vi "PH_Stepmotor_BaseClass.pack PSDB Data.vi"(0 "i ref in":refnum<vi>, 5 "error in (no error)":errorcluster) -> (14 "VI out":refnum<vi>, 15 "PSDB Boolean Data Array":T1[](array[typedef]), 17 "PSDB Numeric Data Array":T3[](array[typedef]), 18 "PSDB String Data Array":T2[](array[typedef]), 19 "error out":errorcluster)   [LabVIEW 2014, in "PH_Stepmotor_BaseClass.lvlib"]
uses:
  PH_Stepmotor_BaseClass.lvlib
  PH_Stepmotor_BaseClass.Motor Type.ctl
  PH_PSDBWriter/PH_PSDBWriter.Numeric dataset.ctl
  PH_PSDBWriter/PH_PSDBWriter.String dataset.ctl
  PH_PSDBWriter/PH_PSDBWriter.Boolean dataset.ctl
  PH_PSDBWriter/PH_PSDBWriter.lvlib
panel:
  in  "SW Scale.Motor Type":T4
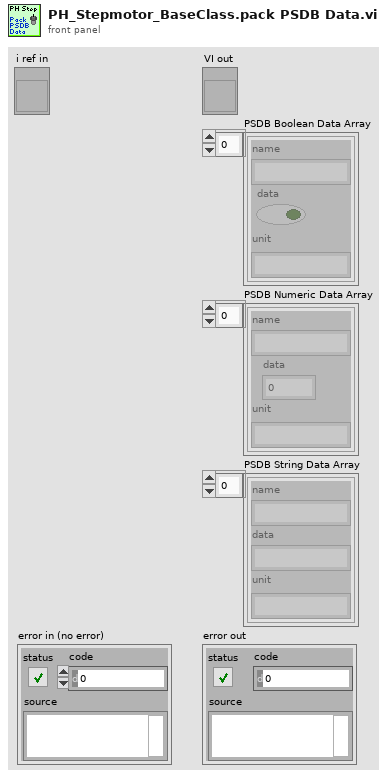
[diagram p1: front panel]
types:
  T1 = typedef "PH_PSDBWriter.lvlib/PH_PSDBWriter.Boolean dataset.ctl" = cluster{"name":string, "data":bool, "unit":string}
  T2 = typedef "PH_PSDBWriter.lvlib/PH_PSDBWriter.String dataset.ctl" = cluster{"name":string, "data":string, "unit":string}
  T3 = typedef "PH_PSDBWriter.lvlib/PH_PSDBWriter.Numeric dataset.ctl" = cluster{"name":string, "data":dbl, "unit":string}
  T4 = typedef "PH_Stepmotor_BaseClass.lvlib/PH_Stepmotor_BaseClass.Motor Type.ctl" = enum16{"Unspecific", "OWIS 49.120.2633", "OWIS 49.060.1033", "OWIS 43.040.2558", "Diamond Motion 2200 series", "OWIS 49.120.266B.MV6", "Calorimeter", "Linear Stage 1", "MICOS VT-80", "MICOS VT-80 S", "Standa Rotstage nt0.95A", "PUF RA 320.200", "PUF RA 800.200", "PUF RA 800.400", "PUF RA 400.50", "1324.nn.800.50", "1324.n9c.800.50", "1324.nn.320.200", "1324.nn.400.200", "1324.nn.800.200", "1324.nn.400.50", "1324.8c9c.800.50", "1324.8c9c.400.200"}
  T5 = typedef "PH_Stepmotor_BaseClass.lvlib/PH_Stepmotor_BaseClass.i attribute.ctl" = cluster{"Device Error":errorcluster, "Axes PSDB Thread":cluster{"Ref":refnum<vi>, "Q-Ref":refnum<queue>, "Data Status":T6}, "Axes":T7[], "Axes PSDB Infos":cluster{"GUI Name":string, "PSDB Instance ID":i32, "PSDB Status Service ID":i32, "Axis":i32, "Class":string}[], "GUI Refs":T11}
  T6 = typedef "PH_PSDBWriter.lvlib/PH_PSDBWriter.Data Status.ctl" = i16
  T7 = typedef "PH_Stepmotor_BaseClass.lvlib/PH_Stepmotor_BaseClass.Axis Attributes.ctl" = cluster{"Settings":T8, "Endswitch?":bool, "DIM Service IDs":T9, "Activity":T10, "Configured?":bool, "Position":cluster{"Current":i32, "Target":i32}, "Position to set":cluster{"New?":bool, "Wanted":i32}, "Stop?":bool, "Reset?":bool, "Move?":bool, "Nothing connected?":bool}
  T8 = typedef "PH_Stepmotor_BaseClass.lvlib/PH_Stepmotor_BaseClass.Axis Settings.ctl" = cluster{"Sign change":bool, "Width":dbl, "Calibration":dbl, "Unit":string, "Motor Type":T4, "Unit Width":string, "Unit CF":string}
  T9 = typedef "PH_Stepmotor_BaseClass.lvlib/PH_Stepmotor_BaseClass.Axis DIM Service IDs.ctl" = cluster{"Settings":i32, "Information":i32}
  T10 = typedef "PH_Stepmotor_BaseClass.lvlib/PH_Stepmotor_BaseClass.Axis Activity.ctl" = enum16{"No Information", "stopped", "running", "Failure", "Alarm", "stopped at backward ES", "stopped at foreward ES"}
  T11 = typedef "PH_Stepmotor_BaseClass.lvlib/PH_Stepmotor_BaseClass.GUI Refs.ctl" = cluster{"Axes Configuration":refnum<vi>, "Device Error":refnum<vi>, "Axes PSDB Infos":refnum<vi>}
  T12 = cluster{"GUI Name":string, "PSDB Instance ID":i32, "PSDB Status Service ID":i32, "Axis":i32, "Class":string}[]
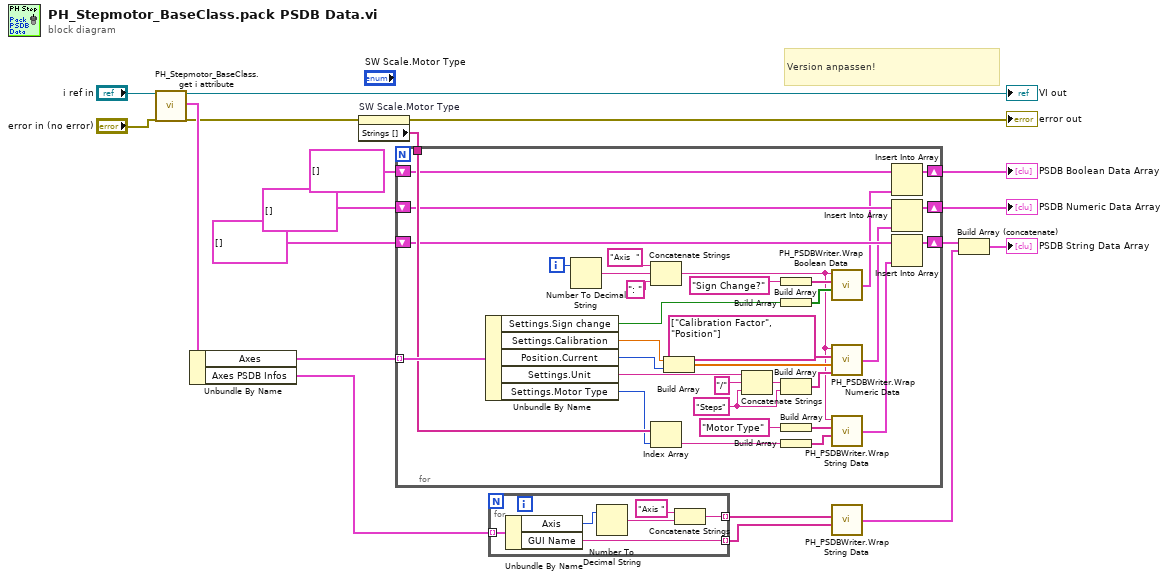
[diagram p0: block diagram]
diagram:
  # "Version anpassen!"
  n1 = call "PH_Stepmotor_BaseClass.get i attribute.vi"("i ref in"="i ref in", "error in (no error)"="error in (no error)") -> ("i ref out"=→"VI out":refnum<vi>, "i attribute"=w9:T5, "error out"=w3:errorcluster)  [unwired: 15 in]
  n2 = Unbundle By Name(w9) -> ("Axes"=w11:T7[], "Axes PSDB Infos"=w10:T12)
  n3 = property on="SW Scale.Motor Type" class="Enum (strict)"(error in=w3) -> (error out=→"error out":errorcluster, "Strings []"=w1:string[])  [unwired: 1 in, 1 out]
  n4 = for {
    tunnel: w11 -> [w53] mode=indexing
    tunnel: w1 -> [w52]
    shift-right: [w50] -> w13
    shift-left: T1[] [] -> [w49]
    shift-right: [w48] -> w16
    shift-left: T3[] [] -> [w47]
    shift-right: [w46] -> w8
    shift-left: T2[] [] -> [w45]
    i -> [w44]
    w36 = "Steps" ("string")
    n5 = Unbundle By Name(w53) -> ("Settings.Sign change"=w34:bool, "Settings.Calibration"=w41:dbl, "Position.Current"=w40:i32, "Settings.Unit"=w37:string, "Settings.Motor Type"=w39:T4)
    n6 = Number To Decimal String(number=w44) -> (decimal integer string=w43:string)  [unwired: 1 in]
    n7 = Concatenate Strings("Axis  ", w43, ": " ("string")) -> (w21:string)
    n8 = Index Array(array=w52, index=w39) -> (element=w30:string)
    n9 = Build Array(w41, w40) -> (w24:dbl[])
    n10 = Concatenate Strings(w37, "/" ("string"), w36) -> (w38:string)
    n11 = Build Array("Sign Change?") -> (w32:string[])
    n12 = Build Array(w34) -> (w33:bool[])
    n13 = Build Array(w38, w36) -> (w25:string[])
    n14 = Build Array("Motor Type") -> (w29:string[])
    n15 = Build Array(w30) -> (w28:string[])
    n16 = call "PH_PSDBWriter.Wrap Boolean Data.vi"("Data Array"=w33, "Name Array"=w32, "Name Prefix"=w21) -> ("PSDB Boolean Data Array"=w31:T1[])  [unwired: 1 in]
    n17 = call "PH_PSDBWriter.Wrap Numeric Data.vi"("Unit Array"=w25, "Data Array"=w24, "Name Array"=string[] ["Calibration Factor", "Position"], "Name Prefix"=w21) -> ("PSDB Numeric Data Array"=w26:T3[])
    n18 = call "PH_PSDBWriter.Wrap String Data.vi"("Data Array"=w28, "Name Array"=w29, "Name Prefix"=w21) -> ("PSDB String Data Array"=w27:T2[])  [unwired: 1 in]
    n19 = Insert Into Array(array=w49, new element=w31) -> (w50:T1[])  [unwired: 1 in]
    n20 = Insert Into Array(array=w47, new element=w26) -> (w48:T3[])  [unwired: 1 in]
    n21 = Insert Into Array(array=w45, new element=w27) -> (w46:T2[])  [unwired: 1 in]
  }
  "PSDB Numeric Data Array" <- w16
  "PSDB Boolean Data Array" <- w13
  n22 = for {
    tunnel: w10 -> [w57] mode=indexing
    tunnel: [w55] -> w19 mode=indexing
    tunnel: [w58] -> w18 mode=indexing
    n23 = Unbundle By Name(w57) -> ("Axis"=w54:i32, "GUI Name"=w55:string)
    n24 = Number To Decimal String(number=w54) -> (decimal integer string=w56:string)  [unwired: 1 in]
    n25 = Concatenate Strings("Axis ", w56) -> (w58:string)
  }
  n26 = call "PH_PSDBWriter.Wrap String Data.vi"("Data Array"=w19, "Name Array"=w18) -> ("PSDB String Data Array"=w15:T2[])  [unwired: 2 in]
  n27 = Build Array (concatenate)(w8, w15) -> (→"PSDB String Data Array":T2[])
